vi "外设配置对话框.vi"() -> ()   [LabVIEW 2016, in "斯坦道氨氮.lvlib"]
uses:
  <vilib>/Utility/miscctls.llb/LVPointTypeDef.ctl
panel:
  out "外设参数选择":enum32{"V3.1版", "V4版", "V3版", "V4.2版"}(tab)
  in  "V3.1版外设配置":T1 {"阀方向" items=["顺时针", "逆时针", "就近"]; "总氮x公式0" items=["0", "1"]; "光谱仪类型" items=["1型", "2型", "3型", "2型氙灯联控"]; "泵阀量" items=["9通"=9, "10通"=10, "12通"=12]; "泵类型" items=["1型", "2型", "sy04型+旋转阀"]}
  in  "v4版外设配置":T2 {"阀型号" items=["垦拓10通阀"]; "总氮x公式0" items=["0", "1"]; "光谱仪类型" items=["1型", "2型", "3型", "2型氙灯联控"]; "泵类型" items=["润泽注射泵", "垦拓注射泵"]}
  in  "V3版外设配置":T3 {"总氮x公式0" items=["0", "1"]; "光谱仪类型" items=["1型", "2型", "3型", "2型氙灯联控"]; "泵阀量" items=["9通"=9, "10通"=10, "12通"=12]; "泵类型" items=["1型", "2型", "sy04型+旋转阀"]}
  in  "v4.2外设配置":T4 {"工作模式" items=["受控模式", "自主模式", "维护模式"]; "阀型号" items=["垦拓10通阀"]; "总氮x公式0" items=["0", "1"]; "光谱仪类型" items=["1型", "1型氙灯联控"]; "泵类型" items=["润泽注射泵", "垦拓注射泵"]}
  in  "关闭":bool
  in  "保存":bool
  in  "读取":bool
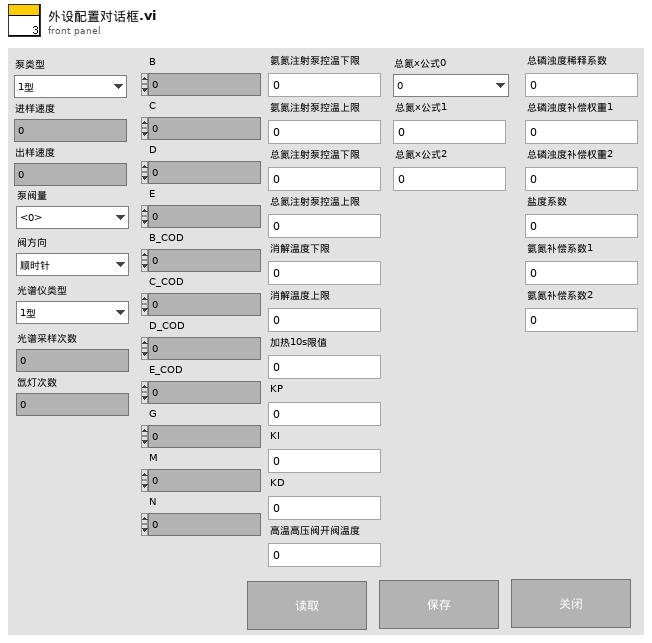
[diagram p1: front panel]
types:
  T1 = typedef "斯坦道氨氮.lvlib/V3.1版外设参数.ctl" = cluster{"泵类型":u8, "进样速度":u32, "出样速度":u32, "泵阀量":u8, "阀方向":u8, "光谱仪类型":u8, "光谱采样次数":u8, "氙灯次数":u8, "B":u16, "C":u16, "D":u16, "E":u16, "B_COD":u16, "C_COD":u16, "D_COD":u16, "E_COD":u16, "G":u16, "M":u16, "N":u16, "氨氮注射泵控温下限":sgl, "氨氮注射泵控温上限":sgl, "总氮注射泵控温下限":sgl, "总氮注射泵控温上限":sgl, "消解温度下限":sgl, "消解温度上限":sgl, "加热10s限值":sgl, "KP":sgl, "KI":sgl, "KD":sgl, "高温高压阀开阀温度":sgl, "总氮x公式0":u8, "总氮x公式1":sgl, "总氮x公式2":sgl, "总磷浊度稀释系数":sgl, "总磷浊度补偿权重1":sgl, "总磷浊度补偿权重2":sgl, "盐度系数":sgl, "氨氮补偿系数1":sgl, "氨氮补偿系数2":sgl}
  T2 = typedef "斯坦道氨氮.lvlib/V4版外设参数.ctl" = cluster{"泵类型":u8, "注射泵正常速度":u32, "注射泵慢速":u32, "阀型号":u8, "res":u8, "光谱仪类型":u8, "光谱采样次数":u8, "氙灯次数":u8, "B":u16, "C":u16, "D":u16, "E":u16, "B_COD":u16, "C_COD":u16, "D_COD":u16, "E_COD":u16, "G":u16, "M":u16, "N":u16, "降温下限":sgl, "降温上限":sgl, "恒温温度下限":sgl, "恒温温度上限":sgl, "消解温度下限":sgl, "消解温度上限":sgl, "加热10s限值":sgl, "KP":sgl, "KI":sgl, "KD":sgl, "高温高压阀开阀温度":sgl, "总氮x公式0":u8, "总氮x公式1":sgl, "总氮x公式2":sgl, "总磷浊度稀释系数":sgl, "总磷浊度补偿权重1":sgl, "总磷浊度补偿权重2":sgl, "盐度系数":sgl, "氨氮补偿系数1":sgl, "氨氮补偿系数2":sgl, "缺试剂传感器阈值":u16}
  T3 = typedef "斯坦道氨氮.lvlib/V3版外设参数.ctl" = cluster{"泵类型":u8, "进样速度":u32, "出样速度":u32, "泵阀量":u8, "光谱仪类型":u8, "光谱采样次数":u8, "氙灯次数":u8, "B":u16, "C":u16, "D":u16, "E":u16, "B_COD":u16, "C_COD":u16, "D_COD":u16, "E_COD":u16, "G":u16, "M":u16, "N":u16, "氨氮注射泵控温下限":sgl, "氨氮注射泵控温上限":sgl, "总氮注射泵控温下限":sgl, "总氮注射泵控温上限":sgl, "消解温度下限":sgl, "消解温度上限":sgl, "加热10s限值":sgl, "高温高压阀开阀温度":sgl, "总氮x公式0":u8, "总氮x公式1":sgl, "总氮x公式2":sgl, "总磷浊度稀释系数":sgl, "总磷浊度补偿权重1":sgl, "总磷浊度补偿权重2":sgl, "盐度系数":sgl, "氨氮补偿系数1":sgl, "氨氮补偿系数2":sgl}
  T4 = typedef "斯坦道氨氮.lvlib/V4.2版外设参数.ctl" = cluster{"工作模式":u16, "泵类型":u16, "阀型号":u16, "注射泵进样速度":u16, "注射泵出样速度":u16, "注射泵滴定速度":u16, "res":u16, "注射泵慢速":u16, "光谱仪类型":u16, "光谱采样次数":u16, "氙灯次数":u16, "B":u16, "C":u16, "D":u16, "E":u16, "B_COD":u16, "C_COD":u16, "D_COD":u16, "E_COD":u16, "G":u16, "M":u16, "N":u16, "温度校准参数":sgl, "降温温度":sgl, "恒温温度":sgl, "消解温度":sgl, "高温高压阀开阀温度":sgl, "加热超时时间":sgl, "KP":sgl, "KI":sgl, "KD":sgl, "消解PID积分上限":sgl, "恒温PID积分上限":sgl, "PID积分下限":sgl, "缺试剂传感器阈值":u16, "滴定延时":u16, "滴定斜率阈值":sgl, "总氮x公式0":u16, "总氮x公式1":sgl, "总氮x公式2":sgl, "总磷浊度稀释系数":sgl, "总磷浊度补偿权重1":sgl, "总磷浊度补偿权重2":sgl, "盐度系数":sgl, "氨氮补偿系数1":sgl, "氨氮补偿系数2":sgl}
  T5 = typedef "LVPointTypeDef.ctl" = cluster{"Horizontal":i16, "Vertical":i16}
  T6 = typedef "SingleStepTestV3.lvlib/SingleStepTestV3.lvclass/仪器版本.ctl" = enum16{"V3.1版", "V4版", "V3版", "V4.2版"}
  T7 = typedef "操作日志字段定义.ctl" = cluster{"时间":timestamp, "参数":string, "日志信息":string, "流程参数":string}
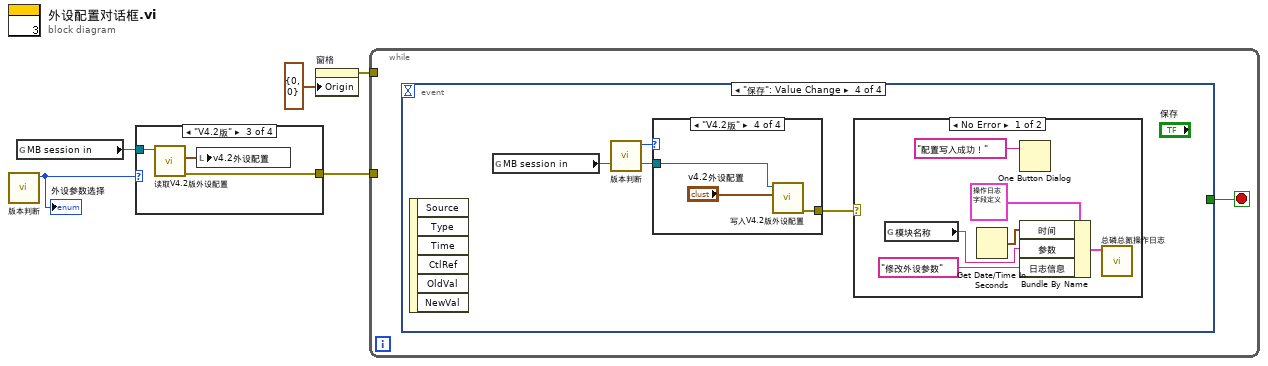
[diagram p0: block diagram]
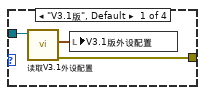
[diagram p2: hidden frame]
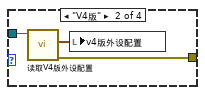
[diagram p3: hidden frame]
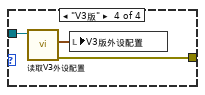
[diagram p4: hidden frame]
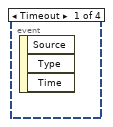
[diagram p5: hidden frame]
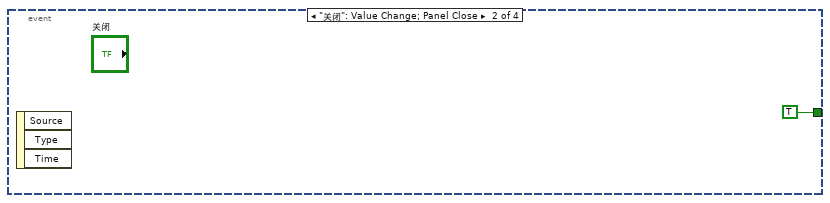
[diagram p6: hidden frame]
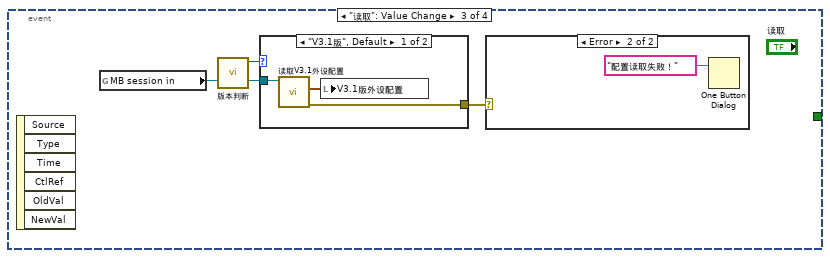
[diagram p7: hidden frame]
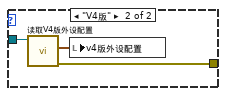
[diagram p9: hidden frame]
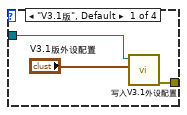
[diagram p11: hidden frame]
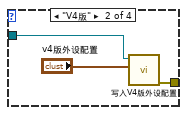
[diagram p12: hidden frame]
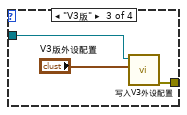
[diagram p13: hidden frame]
diagram:
  n1 = call "版本判断.vi"() -> ("仪器版本"=w1:T6)  [unwired: 11 in]
  "外设参数选择" <- w1
  n2 = global read "VAR总磷总氮全局变量.vi" "MB session in"() -> (w2:refnum<class "MB_Master.lvclass">)
  n3 = case shown="\"V4.2版\"" w1 {
    tunnel: [w8 w10 w13 w16] -> w5
    tunnel: w2 -> [w6 w11 w14 w17]
    frame "V3.1版", Default {
      n4 = call "读取V3.1外设配置.vi"("MB session in"=w6) -> ("error out"=w8:errorcluster, "外设配置"=w7:T1)  [unwired: 8 in, 1 out]
      n5 = local write "V3.1版外设配置"(w7) -> ()
    }
    frame "V4版" {
      n6 = call "读取V4版外设配置.vi"("MB session in"=w11) -> ("error out"=w10:errorcluster, "外设配置"=w9:T2)  [unwired: 8 in, 1 out]
      n7 = local write "v4版外设配置"(w9) -> ()
    }
    frame "V4.2版" {
      n8 = call "读取V4.2版外设配置.vi"("MB session in"=w14) -> ("error out"=w13:errorcluster, "外设配置"=w12:T4)  [unwired: 8 in, 1 out]
      n9 = local write "v4.2外设配置"(w12) -> ()
    }
    frame "V3版" {
      n10 = call "读取V3外设配置.vi"("MB session in"=w17) -> ("error out"=w16:errorcluster, "外设配置"=w15:T3)  [unwired: 8 in, 1 out]
      n11 = local write "V3版外设配置"(w15) -> ()
    }
  }
  n12 = property on="窗格" class="Pane"("Origin"=T5 {"Horizontal"=0, "Vertical"=0} ("原点")) -> (error out=w3:errorcluster)  [unwired: 2 in, 1 out]
  n13 = while {
    tunnel: w5 -> [_]
    tunnel: w3 -> [_]
    stop <- w18 stop-if-true
    n14 = event shown="[3] \"保存\": Value Change" {
      selector: _ -> [_ _ _ _]
      dyn-events: _ -> [_ _ _ _]
      timeout: _ -> [_ _ _ _]
      tunnel: [_ TRUE _ _] -> w18
      event Timeout {
        n15 = event-data() -> ()  [unwired: 1 in, 3 out]
      }
      event "关闭": Value Change; Panel Close {
        n16 = event-data() -> ()  [unwired: 1 in, 3 out]
      }
      event "读取": Value Change {
        n17 = event-data() -> ()  [unwired: 1 in, 6 out]
        n18 = global read "VAR总磷总氮全局变量.vi" "MB session in"() -> (w21:refnum<class "MB_Master.lvclass">)
        n19 = call "版本判断.vi"() -> ("仪器版本"=w22:T6)  [unwired: 11 in]
        n20 = case shown="\"V3.1版\", Default" w22 {
          tunnel: [w26 w28] -> w20
          tunnel: w21 -> [w24 w29]
          frame "V3.1版", Default {
            n21 = call "读取V3.1外设配置.vi"("MB session in"=w24) -> ("error out"=w26:errorcluster, "外设配置"=w25:T1)  [unwired: 8 in, 1 out]
            n22 = local write "V3.1版外设配置"(w25) -> ()
          }
          frame "V4版" {
            n23 = call "读取V4版外设配置.vi"("MB session in"=w29) -> ("error out"=w28:errorcluster, "外设配置"=w27:T2)  [unwired: 8 in, 1 out]
            n24 = local write "v4版外设配置"(w27) -> ()
          }
        }
        n25 = case shown="Error" w20 {
          frame No Error {
          }
          frame Error {
            n26 = One Button Dialog(message="配置读取失败！") -> ()  [unwired: 1 in, 1 out]
          }
        }
      }
      event "保存": Value Change {
        n27 = event-data() -> ()  [unwired: 1 in, 6 out]
        n28 = global read "VAR总磷总氮全局变量.vi" "MB session in"() -> (w32:refnum<class "MB_Master.lvclass">)
        n29 = call "版本判断.vi"() -> ("仪器版本"=w31:T6)  [unwired: 11 in]
        n30 = case shown="\"V4.2版\"" w31 {
          tunnel: [w41 w42 w46 w49] -> w30
          tunnel: w32 -> [w40 w43 w47 w48]
          frame "V3.1版", Default {
            n31 = call "写入V3.1外设配置.vi"("外设配置"="V3.1版外设配置", "MB session in"=w40) -> ("error out"=w41:errorcluster)  [unwired: 8 in, 1 out]
          }
          frame "V4版" {
            n32 = call "写入V4版外设配置.vi"("外设配置"="v4版外设配置", "MB session in"=w43) -> ("error out"=w42:errorcluster)  [unwired: 8 in, 1 out]
          }
          frame "V3版" {
            n33 = call "写入V3外设配置.vi"("外设配置"="V3版外设配置", "MB session in"=w47) -> ("error out"=w46:errorcluster)  [unwired: 8 in, 1 out]
          }
          frame "V4.2版" {
            n34 = call "写入V4.2版外设配置.vi"("外设配置"="v4.2外设配置", "MB session in"=w48) -> ("error out"=w49:errorcluster)  [unwired: 8 in, 1 out]
          }
        }
        n35 = case shown="No Error" w30 {
          frame No Error {
            n36 = global read "VAR总磷总氮全局变量.vi" "模块名称"() -> (w33:string)
            n37 = Get Date/Time In Seconds() -> (seconds since 1Jan1904=w35:timestamp)
            n38 = One Button Dialog(message="配置写入成功！") -> ()  [unwired: 1 in, 1 out]
            n39 = Bundle By Name(cluster=T7 {"时间"=timestamp(0 s since 1904-01-01), "参数"="", "日志信息"="", "流程参数"=""} ("data in"), "时间"=w35, "参数"=w33, "日志信息"="修改外设参数") -> (w36:T7)
            n40 = call "总磷总氮操作日志.vi"("data in"=w36) -> ()  [unwired: 10 in, 1 out]
          }
          frame Error {
          }
        }
      }
    }
  }
